vi "Pre-Uninstall Custom Action.vi"(10 "Variant":variant) -> (0 "error out":errorcluster)   [LabVIEW 2014]
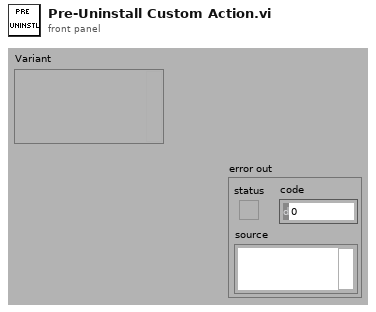
[diagram p1: front panel]
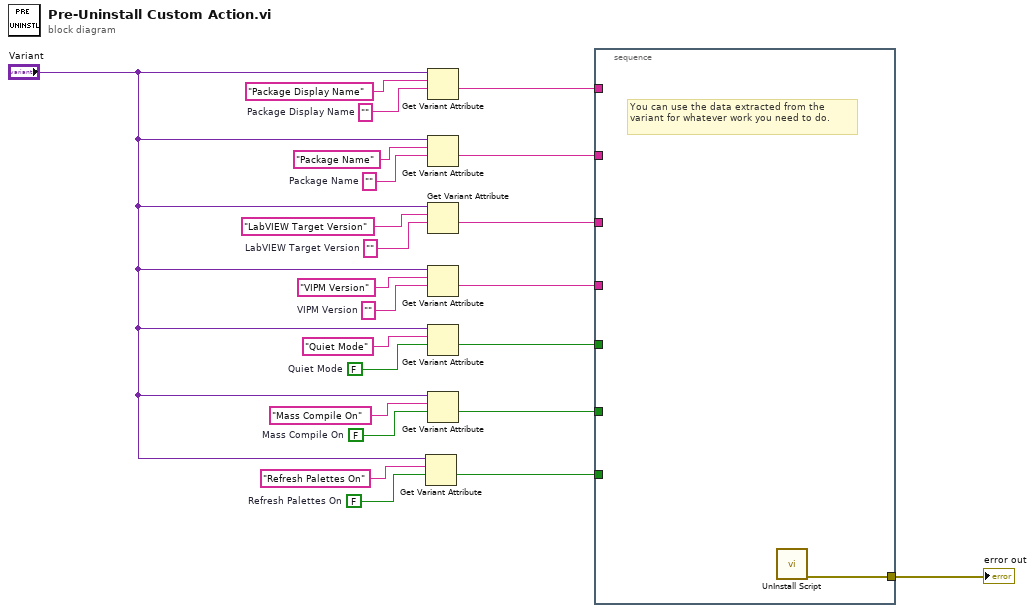
[diagram p0: block diagram]
diagram:
  w2 = FALSE  # Refresh Palettes On
  w3 = FALSE  # Mass Compile On
  w7 = ""  # Package Display Name
  w14 = FALSE  # Quiet Mode
  w17 = ""  # VIPM Version
  w19 = ""  # LabVIEW Target Version
  w21 = ""  # Package Name
  n1 = Get Variant Attribute(Variant="Variant", name="Refresh Palettes On", default value (empty Variant)=w2) -> (value=w6:bool)  [unwired: 1 in, 3 out]
  n2 = Get Variant Attribute(Variant="Variant", name="Package Display Name", default value (empty Variant)=w7) -> (value=w13:string)  [unwired: 1 in, 3 out]
  n3 = Get Variant Attribute(Variant="Variant", name="Package Name", default value (empty Variant)=w21) -> (value=w12:string)  [unwired: 1 in, 3 out]
  n4 = Get Variant Attribute(Variant="Variant", name="LabVIEW Target Version", default value (empty Variant)=w19) -> (value=w11:string)  [unwired: 1 in, 3 out]
  n5 = Get Variant Attribute(Variant="Variant", name="VIPM Version", default value (empty Variant)=w17) -> (value=w10:string)  [unwired: 1 in, 3 out]
  n6 = Get Variant Attribute(Variant="Variant", name="Quiet Mode", default value (empty Variant)=w14) -> (value=w9:bool)  [unwired: 1 in, 3 out]
  n7 = Get Variant Attribute(Variant="Variant", name="Mass Compile On", default value (empty Variant)=w3) -> (value=w8:bool)  [unwired: 1 in, 3 out]
  n8 = stacked-sequence {
    tunnel: w13 -> [_]
    tunnel: w12 -> [_]
    tunnel: w11 -> [_]
    tunnel: w10 -> [_]
    tunnel: w9 -> [_]
    tunnel: w8 -> [_]
    tunnel: w6 -> [_]
    tunnel: [w24] -> w1
    frame #0 {
      # "You can use the data extracted from the variant for whatever work you need to do."
      n9 = call "UnInstall Script.vi"() -> ("error out"=w24:errorcluster)  [unwired: 11 in]
    }
  }
  "error out" <- w1
